vi "Actor Core.vi"(8 "error in":errorcluster, 11 "TestSetup in":refnum<class "TestSetup.lvclass">) -> (0 "error out":errorcluster, 3 "Actor out":refnum<class "Actor.lvclass">)   [LabVIEW 2019, in "TestSetup.lvlib" / "TestSetup.lvclass"]
doc: "(<B>Filename</B>: Actor Framework.lvlib:Actor.lvclass:Actor Core.vi)\n\nReceives messages to the actor, reacts to them, and initiates any error handling that may shut the actor down.\n\nDescendant classes may override this VI to append parallel tasks for the actor to complete while it handles messages. Overrides use the Call Parent Method node."
uses:
  TestSetup.lvclass
  C:/Program Files (x86)/National Instruments/LabVIEW 2019/vi.lib/ActorFramework/Actor/Actor.lvclass
  <vilib>/ActorFramework/Actor/Actor.lvclass
  TestSetup.lvclass/TestSetup.ctl
  <vilib>/ActorFramework/Actor/Actor.lvclass/Actor.ctl
  <vilib>/ActorFramework/Message Enqueuer/Message Enqueuer.lvclass/Message Enqueuer.ctl
  TestSetup Messages/LimitSetting Msg/LimitSetting Msg.lvclass/LimitSetting Msg.ctl
  226a1422-65c0-414f-be6e-00db8bf823a7.vi
  <vilib>/ActorFramework/Message Enqueuer/Init from Existing Queue.vi
  <vilib>/ActorFramework/Message Enqueuer/Enqueue.vi
  SystemSetup/SystemSetup Messages/RefreshSystemConfigurationUI Msg/RefreshSystemConfigurationUI Msg.lvclass
  C:/Program Files (x86)/National Instruments/LabVIEW 2019/vi.lib/ActorFramework/Message/Message.lvclass
  SystemSetup/SystemSetup Messages/SaveSystemConfigurationUI Msg/SaveSystemConfigurationUI Msg.lvclass
  TestSetup Messages/LimitSetting Msg/LimitSetting Msg.lvclass
  <vilib>/ActorFramework/Message Priority Queue/Priority Enqueue.vi
  <vilib>/ActorFramework/Message Enqueuer/Message Enqueuer.lvclass
  SystemSetup/SystemSetup/SystemSetup.lvclass
panel:
  in  "Multicolumn Listbox":i32(listbox)
  in  "Refresh":bool
  in  "TestLimitPath":path
  in  "Save":bool
  in  "Cancel":bool
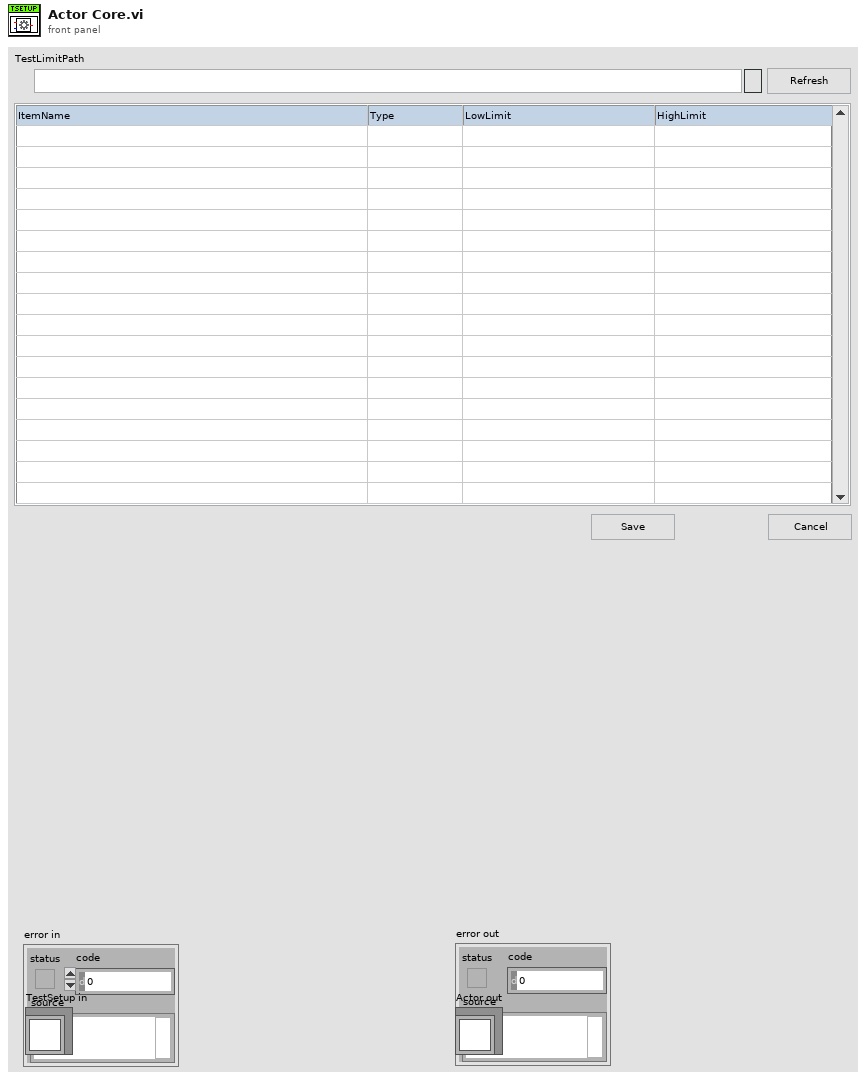
[diagram p1: front panel]
types:
  T1 = enum32{"existing file", "new file", "new or existing file", "existing dir", "new dir", "new or existing dir", "existing file (use LLBs)", "new file (use LLBs)", "new or existing file (use LLBs)", "new or existing file or directory (use LLBs)", "existing dir (use LLBs)", "new dir (use LLBs)", "new or existing dir (use LLBs)", "existing file or dir", "new file or dir", "new or existing file or dir", "existing file or dir (use LLBs)", "new file or dir (use LLBs)"}
  T2 = enum32{"Invalid", "Standard", "Closed", "Hidden", "Minimized", "Maximized"}
  T3 = enum32{"invalid app kind", "Development System", "Run Time System", "Student Edition", "Embedded LabVIEW", "Evaluation", "Custom"}
  T4 = cluster{"Core":cluster{"Current VI Reference":refnum<vi>, "Close Panel on Exit?":bool}, "Your Boolean data":bool, "Your string data":string}
  T5 = cluster{"Current VI Reference":refnum<vi>, "Close Panel on Exit?":bool}
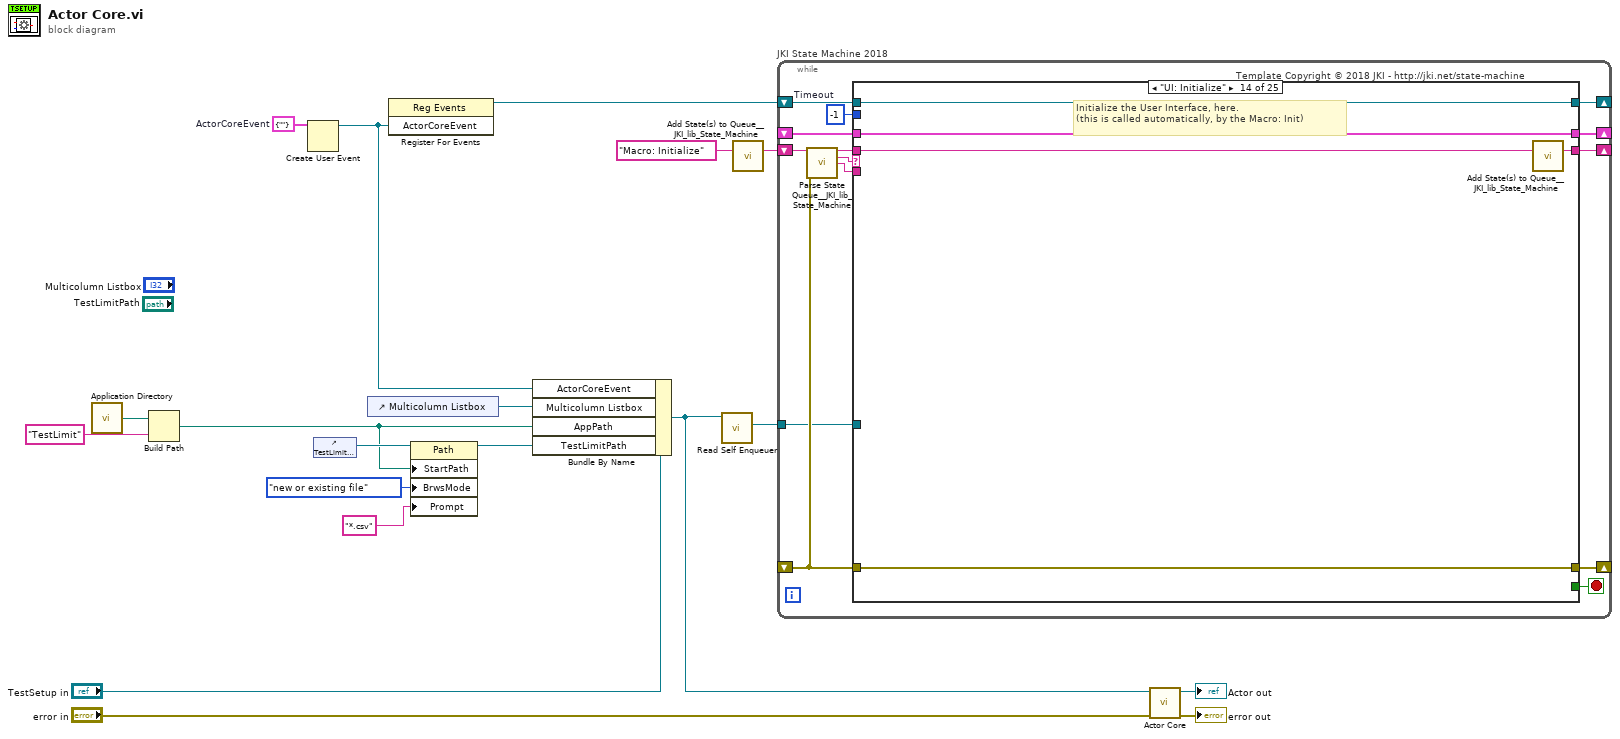
[diagram p0: block diagram]
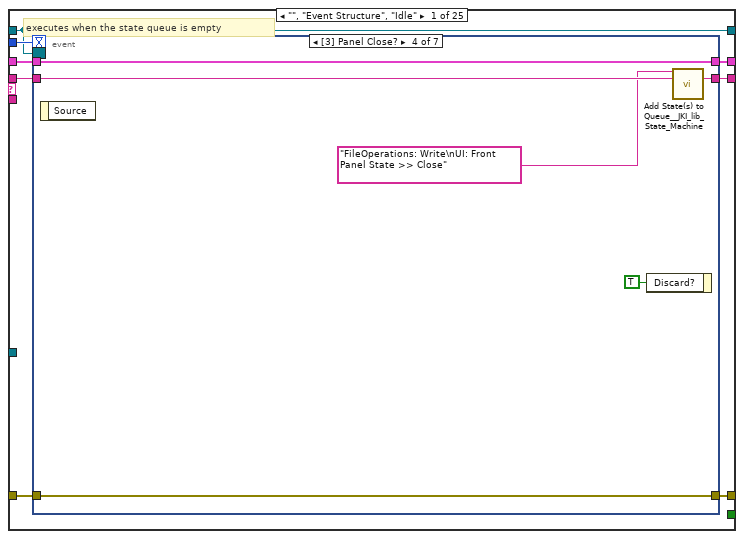
[diagram p2: hidden frame]
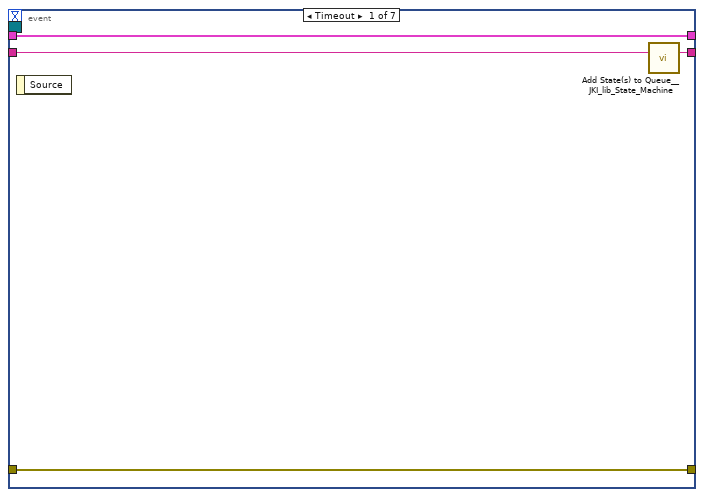
[diagram p3: hidden frame]
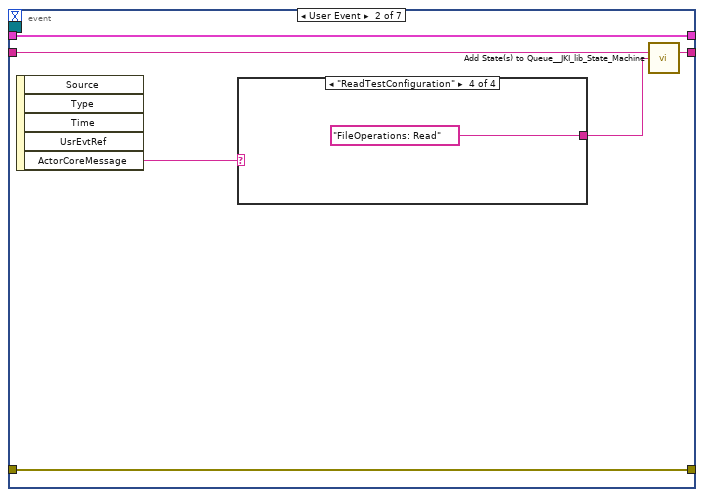
[diagram p4: hidden frame]
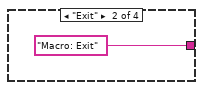
[diagram p6: hidden frame]
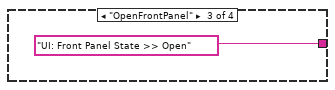
[diagram p7: hidden frame]
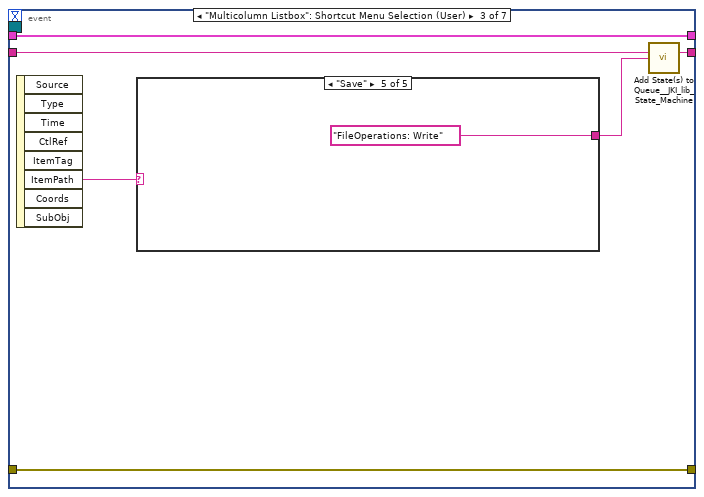
[diagram p8: hidden frame]
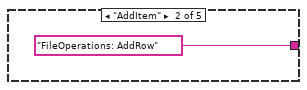
[diagram p10: hidden frame]
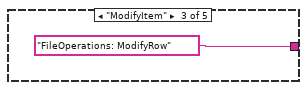
[diagram p11: hidden frame]
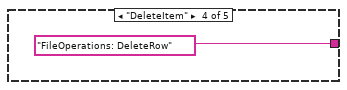
[diagram p12: hidden frame]
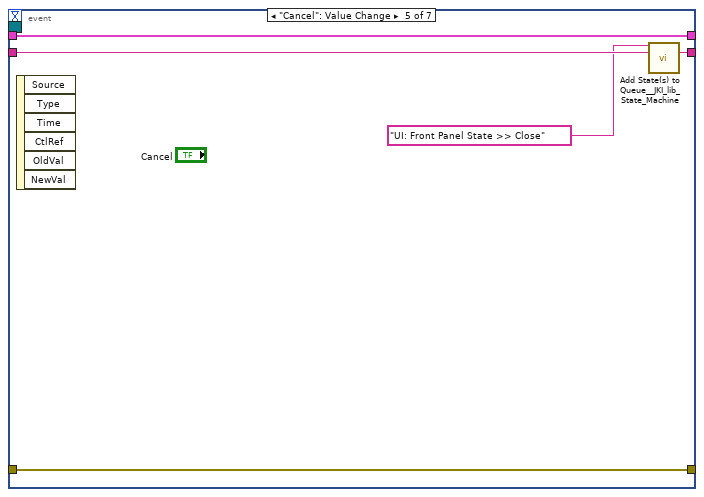
[diagram p13: hidden frame]
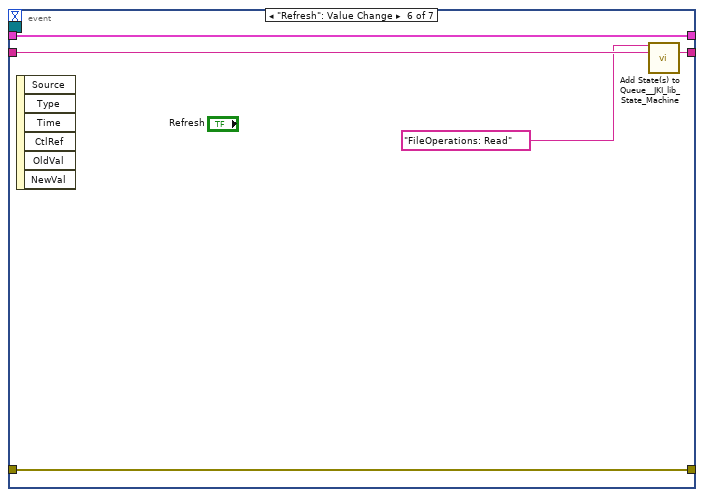
[diagram p14: hidden frame]
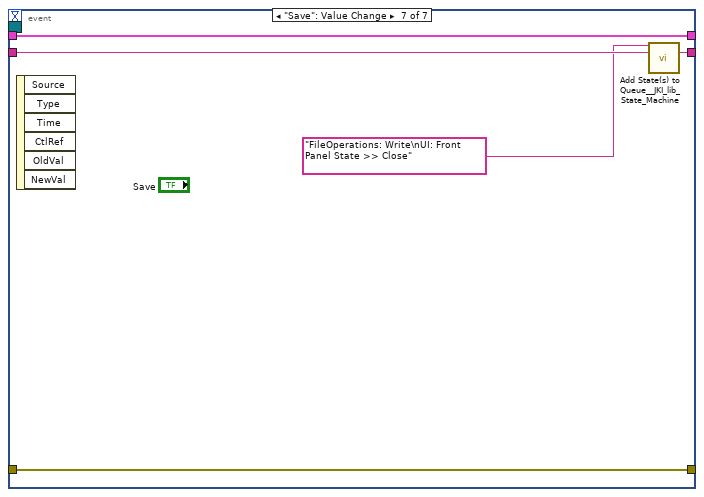
[diagram p15: hidden frame]
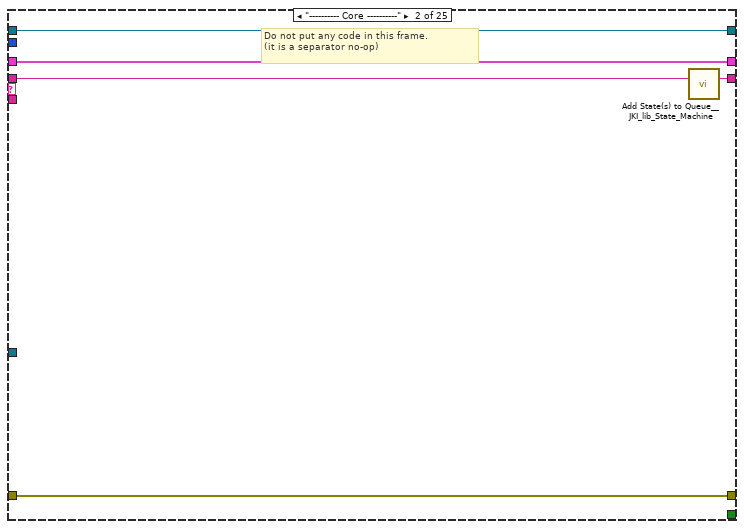
[diagram p16: hidden frame]
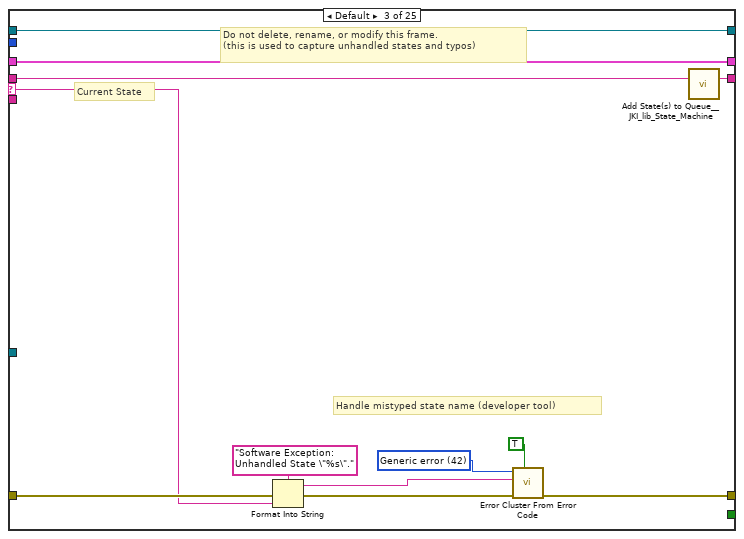
[diagram p17: hidden frame]
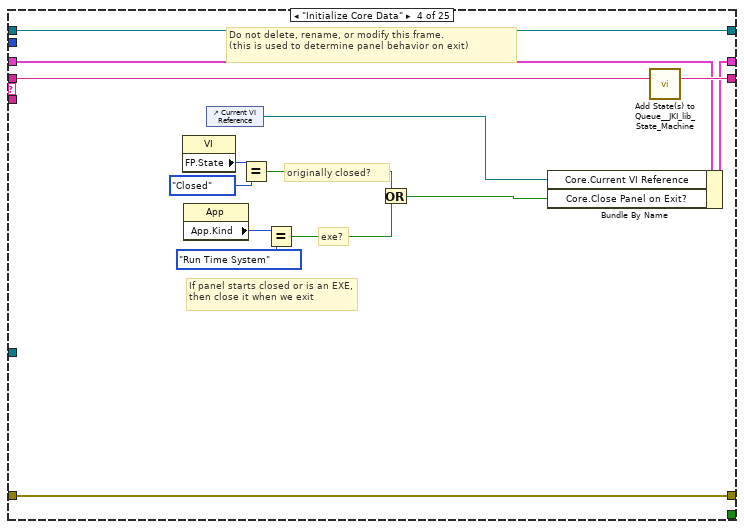
[diagram p18: hidden frame]
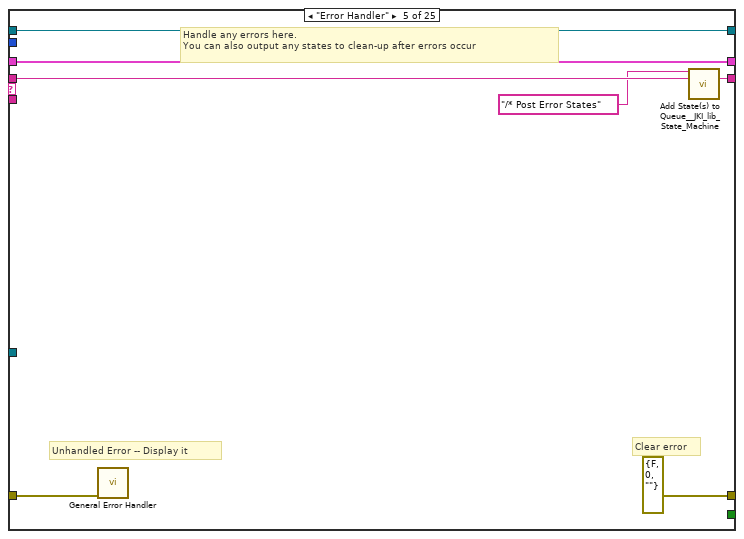
[diagram p19: hidden frame]
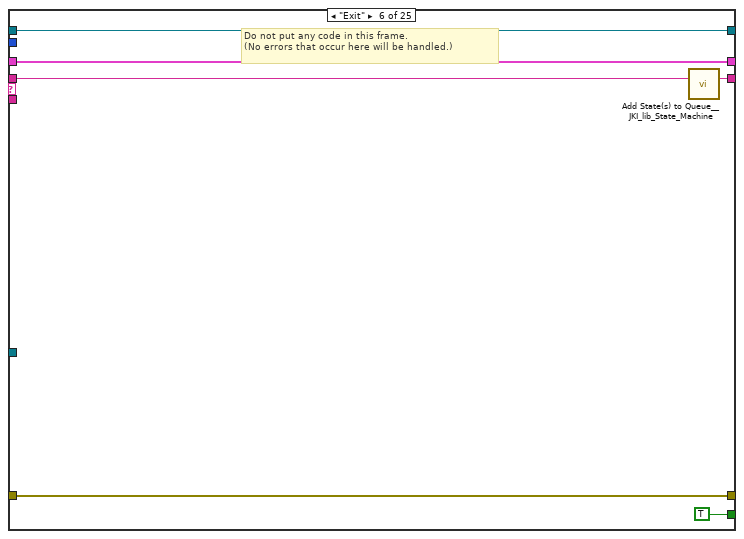
[diagram p20: hidden frame]
diagram:
  w13 = cluster{"ActorCoreMessage":string} {"ActorCoreMessage"=""}  # ActorCoreEvent
  n1 = call <vilib>:"Application Directory.vi"() -> ("Application Directory"=w7:path)
  n2 = Build Path(base path=w7, name or relative path="TestLimit") -> (appended path=w4:path)
  n3 = Create User Event(user event datatype=w13) -> (user event=w11:refnum<user-event>)  [unwired: 1 in, 1 out]
  n4 = control-ref of="TestLimitPath"() -> (w6:refnum<vi>)
  n5 = control-ref of="Multicolumn Listbox"() -> (w1:refnum<vi>)
  n6 = register-events(w11) -> (reference out=w14:refnum<event-registration>)  [unwired: 2 in, 1 out]
  n7 = property class="Path"(reference=w6, "StartPath"=w4, "BrwsMode"=T1."new or existing file" ("Browse Options:Selection Mode"), "Prompt"="*.csv" ("Browse Options:Pattern Label")) -> (reference out=w5:refnum<vi>)  [unwired: 1 in, 1 out]
  n8 = Bundle By Name(cluster="TestSetup in", "ActorCoreEvent"=w11, "Multicolumn Listbox"=w1, "AppPath"=w4, "TestLimitPath"=w5) -> (w10:refnum<class "TestSetup.lvclass">)
  n9 = call <vilib>:"Read Self Enqueuer.vi"("Actor"=w10) -> ("Self Enqueuer"=w9:refnum<class "Message Enqueuer.lvclass">)  [unwired: 10 in]
  n10 = call <vilib>:"Add State(s) to Queue__JKI_lib_State_Machine.vi"("State(s) in (\"\")"="Macro: Initialize") -> ("States Out"=w16:string)  [unwired: 14 in]
  n11 = while "JKI State Machine 2018" {
    shift-right: [w26] -> _
    shift-left: _ -> [w25]
    shift-right: [w29] -> _
    shift-left: _ -> [w23]
    shift-right: [w28] -> _
    shift-left: w16 -> [w30]
    shift-right: [w22] -> _
    shift-left: w14 -> [w21]
    tunnel: w9 -> [w20]
    stop <- w27 stop-if-true
    w24 = -1  # Timeout
    # "Template Copyright © 2018 JKI - http://jki.net/state-machine"
    n12 = call <vilib>:"Parse State Queue__JKI_lib_State_Machine.vi"("State Queue"=w30, "Error In (no error)"=w23) -> ("Remaining States"=w32:string, "Current State"=w33:string, "Arguments"=w31:string)  [unwired: 11 in]
    n13 = case shown="\"UI: Initialize\"" w33 {
      selector: w33 -> [_ _ w92 _ _ _ _ _ _ _ _ _ _ _ _ _ _ _ _ _ _ _ _ _ _]
      tunnel: w32 -> [w41 w90 w96 w116 w123 w129 w134 w142 w149 w154 w159 w165 w170 w175 w182 w194 w264 w272 w283 w288 w294 w300 w307 w314 w321]
      tunnel: w31 -> [_ _ _ _ _ _ _ _ _ _ _ _ _ _ w177 w188 _ _ _ _ _ _ _ _ _]
      tunnel: w25 -> [w39 w87 w94 w109 w120 w127 w131 _ w144 w151 w157 w163 w167 w172 w180 w190 w261 w269 w280 w285 w290 w296 w303 w310 w317]
      tunnel: [w38 w88 w98 w113 errorcluster {"status"=FALSE, "code"=0, "source"=""} ("error out") w126 w132 w139 w145 w152 w156 w160 w168 w171 w178 w191 w262 w266 w281 w286 w292 w298 w305 w312 w319] -> w29
      tunnel: w23 -> [w37 w88 w97 w113 w119 w126 w132 w139 w146 w152 w156 w161 w168 w171 w179 w192 w262 w270 w281 w286 w292 w298 w305 w312 w319]
      tunnel: [w40 w89 w95 w115 w122 w128 w133 w141 w148 w153 w158 w164 w169 w174 w181 w193 w263 w271 w282 w287 w293 w299 w306 w313 w320] -> w28
      tunnel: [_ _ _ _ _ TRUE _ _ _ _ _ _ _ _ _ _ _ _ _ _ _ _ _ _ _] -> w27
      tunnel: [w36 w87 w94 w114 w120 w127 w131 w140 w144 w151 w157 w163 w167 w172 w180 w190 w261 w269 w280 w285 w290 w296 w303 w310 w317] -> w26
      tunnel: w24 -> [w35 _ _ _ _ _ _ _ _ _ _ _ _ _ _ _ _ _ _ _ _ _ _ _ _]
      tunnel: [w34 w86 w91 w103 w117 w124 w130 w135 w143 w150 w155 w162 w166 w173 w176 w187 w260 w267 w273 w284 w291 w297 w304 w311 w318] -> w22
      tunnel: w21 -> [w34 w86 w91 w103 w117 w124 w130 w135 w143 w150 w155 w162 w166 w173 w176 w187 w260 w267 w273 w284 w291 w297 w304 w311 w318]
      tunnel: w20 -> [_ _ _ _ _ _ _ _ _ _ _ _ _ _ _ _ _ _ _ _ w289 w295 w302 w308 w315]
      frame "", "Event Structure", "Idle" {
        # "executes when the state queue is empty"
        n14 = event shown="[3] Panel Close?" {
          selector: w34 -> [_ _ _ _ _ _ _]
          dyn-events: _ -> [_ _ _ _ _ _ _]
          timeout: w35 -> [_ _ _ _ _ _ _]
          tunnel: w41 -> [w45 w51 w60 w70 w75 w80 w85]
          tunnel: [w44 w50 w59 w69 w74 w79 w84] -> w40
          tunnel: w39 -> [w42 w48 w57 w67 w72 w77 w82]
          tunnel: [w43 w49 w58 w68 w73 w78 w83] -> w38
          tunnel: w37 -> [w43 w49 w58 w68 w73 w78 w83]
          tunnel: [w42 w48 w57 w67 w72 w77 w82] -> w36
          event Timeout {
            n15 = event-data() -> ()  [unwired: 1 in, 1 out]
            n16 = call <vilib>:"Add State(s) to Queue__JKI_lib_State_Machine.vi"("State(s) in (\"\")"=w45) -> ("States Out"=w44:string)  [unwired: 14 in]
          }
          event User Event {
            n17 = event-data() -> ("ActorCoreMessage"=w47:string)  [unwired: 1 in, 4 out]
            n18 = case shown="\"ReadTestConfiguration\"" w47 {
              tunnel: [_ "Macro: Exit" "UI: Front Panel State >> Open" "FileOperations: Read"] -> w46
              frame "Idle", Default {
              }
              frame "Exit" {
              }
              frame "OpenFrontPanel" {
              }
              frame "ReadTestConfiguration" {
              }
            }
            n19 = call <vilib>:"Add State(s) to Queue__JKI_lib_State_Machine.vi"("State(s) in (\"\")"=w51, "State(s) at Back (\"\")"=w46) -> ("States Out"=w50:string)  [unwired: 13 in]
          }
          event "Multicolumn Listbox": Shortcut Menu Selection (User) {
            n20 = event-data() -> ("ItemPath"=w55:string)  [unwired: 1 in, 7 out]
            n21 = case shown="\"Save\"" w55 {
              tunnel: [_ "FileOperations: AddRow" "FileOperations: ModifyRow" "FileOperations: DeleteRow" "FileOperations: Write"] -> w56
              frame "Idle", Default {
              }
              frame "AddItem" {
              }
              frame "ModifyItem" {
              }
              frame "DeleteItem" {
              }
              frame "Save" {
              }
            }
            n22 = call <vilib>:"Add State(s) to Queue__JKI_lib_State_Machine.vi"("State(s) in (\"\")"=w60, "State(s) at Back (\"\")"=w56) -> ("States Out"=w59:string)  [unwired: 13 in]
          }
          event Panel Close? {
            n23 = event-data() -> ()  [unwired: 1 in, 1 out]
            n24 = event-data("Discard?"=TRUE) -> ()  [unwired: 1 in, 1 out]
            n25 = call <vilib>:"Add State(s) to Queue__JKI_lib_State_Machine.vi"("State(s) in Front (\"\")"="FileOperations: Write\nUI: Front Panel State >> Close", "State(s) in (\"\")"=w70) -> ("States Out"=w69:string)  [unwired: 13 in]
          }
          event "Cancel": Value Change {
            n26 = event-data() -> ()  [unwired: 1 in, 6 out]
            n27 = call <vilib>:"Add State(s) to Queue__JKI_lib_State_Machine.vi"("State(s) in Front (\"\")"="UI: Front Panel State >> Close", "State(s) in (\"\")"=w75) -> ("States Out"=w74:string)  [unwired: 13 in]
          }
          event "Refresh": Value Change {
            n28 = event-data() -> ()  [unwired: 1 in, 6 out]
            n29 = call <vilib>:"Add State(s) to Queue__JKI_lib_State_Machine.vi"("State(s) in Front (\"\")"="FileOperations: Read", "State(s) in (\"\")"=w80) -> ("States Out"=w79:string)  [unwired: 13 in]
          }
          event "Save": Value Change {
            n30 = event-data() -> ()  [unwired: 1 in, 6 out]
            n31 = call <vilib>:"Add State(s) to Queue__JKI_lib_State_Machine.vi"("State(s) in Front (\"\")"="FileOperations: Write\nUI: Front Panel State >> Close", "State(s) in (\"\")"=w85) -> ("States Out"=w84:string)  [unwired: 13 in]
          }
        }
      }
      frame "---------- Core ----------" {
        # "Do not put any code in this frame.\n(it is a separator no-op)"
        n32 = call <vilib>:"Add State(s) to Queue__JKI_lib_State_Machine.vi"("State(s) in (\"\")"=w90) -> ("States Out"=w89:string)  [unwired: 14 in]
      }
      frame Default {
        w101 = 42 items=["No error", "Argument error", "Memory is full", "Out of zone", "End of file", "File already open", "Generic file I/O error", "File not found", "File permission error", "Disk is full", "Duplicate path", "Too many files open", "System feature not enabled", "Resource file not found", "Cannot add resource", "Resource not found", "Image not found", "Image memory error", "Pen does not exist", "Config type invalid", "Config token not found", "Config parse error", "Config memory error", "Bad external code format", "Bad external code offset", "External code not present", "Null window", "Destroy window error", "Null menu", "Print aborted", "Bad print record", "Print driver error", "Windows error during printing", "Memory error during printing", "Print dialog error", "Generic print error", "Invalid device refnum", "Device not found", "Device parameter error", "Device unit error", "Cannot open device", "Device call aborted", "Generic error", "Cancelled by user", "Object ID too low", "Object ID too high", "Object not in heap", "Unknown heap", "Unknown object (invalid DefProc)", "Unknown object (DefProc not in table)", "Message out of range", "Invalid (null) method", "Unknown message", "Manager call not supported", "Bad address", "Network operation in progress", "Network operation timed out", "Connection is busy", "Network attribute not supported", "Network error", "Address in use", "System out of memory", "Connection aborted", "Connection refused", "Not connected", "Already connected", "Connection closed", "Initialization error (interapplication manager)", "Bad occurrence", "Wait on unbound occurrence handler", "Occurrence queue overflow", "Datalog type conflict", "Unused", "Unrecognized type (interapplication manager)", "Memory corrupt", "Failed to make temporary DLL", "Old CIN version", "Drag socket not found", "Failed to load drop-object", "Failed to register OLE object", "Failed to release OLE object", "Format specifier type mismatch", "Unknown format specifier", "Too few format specifiers", "Too many format specifiers", "Scan failed", "Newer CIN version", "Error converting to variant", "Runtime menu error", "Password tampered", "Variant attribute not found", "Incompatible variant data type", "Event data is not available", "Event Store is not present", "Occurrence is not found", "Event Queue is not created", "Event info is not available", "Refnum passed is NULL", "Error retrieving Class GUID", "Error retrieving CoClass GUID", "Error retrieving TypeLib GUID.", "Bad built application magic bytes.", "Specific driver is different from the specific driver associated with the Logical Name.", "There is no session opened to the class driver.", "Max Error", "MAX - Error with config objects", "MAX - Error loading configuration", "MAX - Group not supported"]
        # "Current State"
        # "Do not delete, rename, or modify this frame.\n(this is used to capture unhandled states and typos)"
        # "Handle mistyped state name (developer tool)"
        n33 = Format Into String(format string="Software Exception: Unhandled State \"%s\"." ("message"), error in=w97, w92) -> (resulting string=w100:string, error out=w99:errorcluster)  [unwired: 1 in]
        n34 = call <vilib>:"Error Cluster From Error Code.vi"("show call chain? (False)"=TRUE, "error in (no error)"=w99, "error message (\"\")"=w100, "error code (0)"=w101) -> ("error out"=w98:errorcluster)  [unwired: 5 in]
        n35 = call <vilib>:"Add State(s) to Queue__JKI_lib_State_Machine.vi"("State(s) in (\"\")"=w96) -> ("States Out"=w95:string)  [unwired: 14 in]
      }
      frame "Initialize Core Data" {
        # "Do not delete, rename, or modify this frame.\n(this is used to determine panel behavior on exit)"
        # "originally closed?"
        # "exe?"
        # "If panel starts closed or is an EXE, then close it when we exit"
        n36 = property class="VI"() -> ("FP.State"=w106:T2)  [unwired: 2 in, 2 out]
        n37 = property class="App"() -> ("App.Kind"=w112:T3)  [unwired: 2 in, 2 out]
        n38 = control-ref of="Current VI Reference"() -> (w107:refnum<vi>)
        n39 = Equal?(x=w106, y=T2."Closed" ("Front Panel Window:State")) -> (x = y?=w104:bool)
        n40 = Equal?(x=w112, y=T3."Run Time System" ("Application:Kind")) -> (x = y?=w110:bool)
        n41 = Or(x=w104, y=w110) -> (x .or. y?=w108:bool)
        n42 = Bundle By Name(cluster=w109, "Core.Current VI Reference"=w107, "Core.Close Panel on Exit?"=w108) -> (w114:T4)
        n43 = call <vilib>:"Add State(s) to Queue__JKI_lib_State_Machine.vi"("State(s) in (\"\")"=w116) -> ("States Out"=w115:string)  [unwired: 14 in]
      }
      frame "Error Handler" {
        # "Unhandled Error -- Display it"
        # "Handle any errors here.\nYou can also output any states to clean-up after errors occur"
        # "Clear error"
        n44 = call <vilib>:"General Error Handler.vi"("error in (no error)"=w119) -> ()  [unwired: 10 in, 5 out]
        n45 = call <vilib>:"Add State(s) to Queue__JKI_lib_State_Machine.vi"("State(s) in Front (\"\")"="/* Post Error States", "State(s) in (\"\")"=w123) -> ("States Out"=w122:string)  [unwired: 13 in]
      }
      frame "Exit" {
        # "Do not put any code in this frame.\n(No errors that occur here will be handled.)"
        n46 = call <vilib>:"Add State(s) to Queue__JKI_lib_State_Machine.vi"("State(s) in (\"\")"=w129) -> ("States Out"=w128:string)  [unwired: 14 in]
      }
      frame "---------- Data ----------" {
        # "Do not put any code in this frame.\n(It is a separator no-op. You can make a copy of this frame to create a new Data frame)"
        n47 = call <vilib>:"Add State(s) to Queue__JKI_lib_State_Machine.vi"("State(s) in (\"\")"=w134) -> ("States Out"=w133:string)  [unwired: 14 in]
      }
      frame "Data: Initialize" {
        w136 = T5 {"Current VI Reference"=refnum, "Close Panel on Exit?"=FALSE}  # Core
        w138 = TRUE  # Your Boolean data
        w137 = ""  # Your string data
        # "Data names and types of shift register data are defined by this bundle."
        # "Initialize the shift-register data, here.\n(data names are defined by what you wire into the bundle function)"
        n48 = Bundle("Core"=w136, "Your Boolean data"=w138, "Your string data"=w137) -> (w140:T4)  [unwired: 1 in]
        n49 = call <vilib>:"Add State(s) to Queue__JKI_lib_State_Machine.vi"("State(s) in (\"\")"=w142) -> ("States Out"=w141:string)  [unwired: 14 in]
      }
      frame "Data: Cleanup" {
        # "Cleanup any data and references, here.\n(this is called automatically, by the Macro: Exit)"
        n50 = Unbundle By Name(w144) -> ("Core.Current VI Reference"=w147:refnum<vi>)
        n51 = Close Reference(reference=w147, error in (no error)=w146) -> (error out=w145:errorcluster)
        n52 = call <vilib>:"Add State(s) to Queue__JKI_lib_State_Machine.vi"("State(s) in (\"\")"=w149) -> ("States Out"=w148:string)  [unwired: 14 in]
      }
      frame "---------- Events ----------" {
        # "Do not put any code in this frame.\n(It is a separator no-op. You can make a copy of this frame to create a new UI frame)"
        n53 = call <vilib>:"Add State(s) to Queue__JKI_lib_State_Machine.vi"("State(s) in (\"\")"=w154) -> ("States Out"=w153:string)  [unwired: 14 in]
      }
      frame "Events: Register" {
        n54 = call <vilib>:"Add State(s) to Queue__JKI_lib_State_Machine.vi"("State(s) in (\"\")"=w159) -> ("States Out"=w158:string)  [unwired: 14 in]
      }
      frame "Events: Unregister" {
        # "Do not put any code in this frame.\n(It is a separator no-op. You can make a copy of this frame to create a new UI frame)"
        n55 = Unregister For Events(event registration refnum=w162, error in=w161) -> (error out=w160:errorcluster)
        n56 = call <vilib>:"Add State(s) to Queue__JKI_lib_State_Machine.vi"("State(s) in (\"\")"=w165) -> ("States Out"=w164:string)  [unwired: 14 in]
      }
      frame "---------- UI ----------" {
        # "Do not put any code in this frame.\n(It is a separator no-op. You can make a copy of this frame to create a new UI frame)"
        n57 = call <vilib>:"Add State(s) to Queue__JKI_lib_State_Machine.vi"("State(s) in (\"\")"=w170) -> ("States Out"=w169:string)  [unwired: 14 in]
      }
      frame "UI: Initialize" {
        # "Initialize the User Interface, here.\n(this is called automatically, by the Macro: Init)"
        n58 = call <vilib>:"Add State(s) to Queue__JKI_lib_State_Machine.vi"("State(s) in (\"\")"=w175) -> ("States Out"=w174:string)  [unwired: 14 in]
      }
      frame "UI: Cursor Set" {
        # "Argument"
        # "Set and Unset Cursor Busy.\n(Usage: \"UI: Cursor Set >> Busy|Idle\")"
        n59 = case shown="\"Idle\", Default" w177 {
          tunnel: w179 -> [w184 w186]
          tunnel: [w183 w185] -> w178
          frame "Idle", Default {
            n60 = call <vilib>:"Unset Busy.vi"("error in (no error)"=w184) -> ("error out"=w183:errorcluster)  [unwired: 10 in]
          }
          frame "Busy" {
            n61 = call <vilib>:"Set Busy.vi"("error in (no error)"=w186) -> ("error out"=w185:errorcluster)  [unwired: 9 in, 1 out]
          }
        }
        n62 = call <vilib>:"Add State(s) to Queue__JKI_lib_State_Machine.vi"("State(s) in (\"\")"=w182) -> ("States Out"=w181:string)  [unwired: 14 in]
      }
      frame "UI: Front Panel State" {
        # "Argument"
        # "Set Front Panel Open or Closed\n(Usage: \"UI: Front Panel State >> Open|Close\")"
        n63 = Unbundle By Name(w190) -> ("Core.Current VI Reference"=w189:refnum<vi>)
        n64 = case shown="\"Minimize\", \"Minimized\"" w188 {
          tunnel: w192 -> [w200 w215 w226 w239 w252]
          tunnel: [w202 w216 w228 w241 w254] -> w191
          tunnel: w189 -> [w201 w213 w227 w240 w253]
          frame "Open", "Standard", Default {
            w195 = T2."Standard" ("State")
            n65 = property class="VI"(reference=w201, error in=w200) -> (reference out=w198:refnum<vi>, error out=w199:errorcluster, "FP.State"=w197:T2)
            n66 = Not Equal?(x=w197, y=w195) -> (x != y?=w196:bool)
            n67 = case shown="True" w196 {
              tunnel: [w206 w208] -> w202
              tunnel: w199 -> [w205 w208]
              tunnel: w198 -> [w204 _]
              tunnel: w195 -> [w203 _]
              frame True {
                n68 = invoke class="VI" method="FP.Open"(reference=w204, error in=w205, "Activate"=TRUE, "State"=w203) -> (error out=w206:errorcluster)  [unwired: 1 in, 4 out]
              }
              frame False {
              }
            }
          }
          frame "Close", "Closed" {
            n69 = property class="VI"(reference=w213, error in=w215) -> (reference out=w212:refnum<vi>, error out=w214:errorcluster, "FP.State"=w210:T2)
            n70 = Not Equal?(x=w210, y=T2."Closed" ("Front Panel Window:State")) -> (x != y?=w209:bool)
            n71 = case shown="True" w209 {
              tunnel: [w217 w220] -> w216
              tunnel: w214 -> [w217 w219]
              tunnel: w212 -> [_ w218]
              frame False {
              }
              frame True {
                n72 = invoke class="VI" method="FP.Close"(reference=w218, error in=w219) -> (error out=w220:errorcluster)  [unwired: 1 in, 2 out]
              }
            }
          }
          frame "Hidden", "Hide" {
            w221 = T2."Hidden" ("State")
            n73 = property class="VI"(reference=w227, error in=w226) -> (reference out=w224:refnum<vi>, error out=w225:errorcluster, "FP.State"=w223:T2)
            n74 = Not Equal?(x=w223, y=w221) -> (x != y?=w222:bool)
            n75 = case shown="True" w222 {
              tunnel: [w232 w233] -> w228
              tunnel: w225 -> [w231 w233]
              tunnel: w224 -> [w230 _]
              tunnel: w221 -> [w229 _]
              frame True {
                n76 = invoke class="VI" method="FP.Open"(reference=w230, error in=w231, "State"=w229) -> (error out=w232:errorcluster)  [unwired: 2 in, 4 out]
              }
              frame False {
              }
            }
          }
          frame "Minimize", "Minimized" {
            w234 = T2."Minimized" ("State")
            n77 = property class="VI"(reference=w240, error in=w239) -> (reference out=w237:refnum<vi>, error out=w238:errorcluster, "FP.State"=w236:T2)
            n78 = Not Equal?(x=w236, y=w234) -> (x != y?=w235:bool)
            n79 = case shown="True" w235 {
              tunnel: [w245 w246] -> w241
              tunnel: w238 -> [w244 w246]
              tunnel: w237 -> [w243 _]
              tunnel: w234 -> [w242 _]
              frame True {
                n80 = invoke class="VI" method="FP.Open"(reference=w243, error in=w244, "State"=w242) -> (error out=w245:errorcluster)  [unwired: 2 in, 4 out]
              }
              frame False {
              }
            }
          }
          frame "Maximize", "Maximized" {
            w247 = T2."Maximized" ("State")
            n81 = property class="VI"(reference=w253, error in=w252) -> (reference out=w250:refnum<vi>, error out=w251:errorcluster, "FP.State"=w249:T2)
            n82 = Not Equal?(x=w249, y=w247) -> (x != y?=w248:bool)
            n83 = case shown="True" w248 {
              tunnel: [w258 w259] -> w254
              tunnel: w251 -> [w257 w259]
              tunnel: w250 -> [w256 _]
              tunnel: w247 -> [w255 _]
              frame True {
                n84 = invoke class="VI" method="FP.Open"(reference=w256, error in=w257, "State"=w255) -> (error out=w258:errorcluster)  [unwired: 2 in, 4 out]
              }
              frame False {
              }
            }
          }
        }
        n85 = call <vilib>:"Add State(s) to Queue__JKI_lib_State_Machine.vi"("State(s) in (\"\")"=w194) -> ("States Out"=w193:string)  [unwired: 14 in]
      }
      frame "---------- Macro ----------" {
        # "Do not put any code in this frame.\n(It is a separator no-op. You can make a copy of this frame to create a new Macro frame)"
        n86 = call <vilib>:"Add State(s) to Queue__JKI_lib_State_Machine.vi"("State(s) in (\"\")"=w264) -> ("States Out"=w263:string)  [unwired: 14 in]
      }
      frame "Macro: Initialize" {
        # "Initialization Macro\n(This is called once, when the VI starts)"
        n87 = call "Stall Data Flow.vim"("value in"=w270, "milliseconds to wait"=u32 500) -> ("value out"=w266:errorcluster)  [unwired: 1 out]
        n88 = call <vilib>:"Add State(s) to Queue__JKI_lib_State_Machine.vi"("State(s) in Front (\"\")"="Data: Initialize\nInitialize Core Data\nEvents: Register\nUI: Initialize\nUI: Front Panel State >> Close", "State(s) in (\"\")"=w272) -> ("States Out"=w271:string)  [unwired: 13 in]
      }
      frame "Macro: Exit" {
        # "Exit Macro\n(This is called once, when the VI exits)"
        n89 = Unbundle By Name(w280) -> ("Core.Close Panel on Exit?"=w279:bool)
        n90 = Select(t="UI: Front Panel State >> Close", s=w279, f="") -> (s? t:f=w276:string)
        n91 = call <vilib>:"Add State(s) to Queue__JKI_lib_State_Machine.vi"("State(s) in (\"\")"=w276, "State(s) at Back (\"\")"="Data: Cleanup\nEvents: Unregister\nExit") -> ("States Out"=w274:string)  [unwired: 13 in]
        n92 = call <vilib>:"Add State(s) to Queue__JKI_lib_State_Machine.vi"("State(s) in Front (\"\")"=w274, "State(s) in (\"\")"=w283) -> ("States Out"=w282:string)  [unwired: 13 in]
      }
      frame "---------- FileOperations ----------" {
        # "Template Separator\n(You can make a copy of, or modify, this frame)"
        n93 = call <vilib>:"Add State(s) to Queue__JKI_lib_State_Machine.vi"("State(s) in (\"\")"=w288) -> ("States Out"=w287:string)  [unwired: 14 in]
      }
      frame "FileOperations: Read" {
        # "Your code here.\n(You can make a copy of, or modify, this frame)"
        n94 = call "Send RefreshSystemConfigurationUI.vi"("Message Enqueuer"=w289) -> ()  [unwired: 9 in, 2 out]
        n95 = call <vilib>:"Add State(s) to Queue__JKI_lib_State_Machine.vi"("State(s) in (\"\")"=w294) -> ("States Out"=w293:string)  [unwired: 14 in]
      }
      frame "FileOperations: Write" {
        # "Your code here.\n(You can make a copy of, or modify, this frame)"
        n96 = call "Send SaveSystemConfigurationUI.vi"("Message Enqueuer"=w295) -> ()  [unwired: 9 in, 2 out]
        n97 = call <vilib>:"Add State(s) to Queue__JKI_lib_State_Machine.vi"("State(s) in (\"\")"=w300) -> ("States Out"=w299:string)  [unwired: 14 in]
      }
      frame "FileOperations: AddRow" {
        # "Your code here.\n(You can make a copy of, or modify, this frame)"
        n98 = call "Send LimitSetting.vi"("operation"=enum16{"Add", "Delete", "Modify"}."Add", "Message Enqueuer"=w302) -> ()  [unwired: 8 in, 2 out]
        n99 = call <vilib>:"Add State(s) to Queue__JKI_lib_State_Machine.vi"("State(s) in (\"\")"=w307) -> ("States Out"=w306:string)  [unwired: 14 in]
      }
      frame "FileOperations: ModifyRow" {
        # "Your code here.\n(You can make a copy of, or modify, this frame)"
        n100 = call "Send LimitSetting.vi"("operation"=enum16{"Add", "Delete", "Modify"}."Modify", "Message Enqueuer"=w308) -> ()  [unwired: 8 in, 2 out]
        n101 = call <vilib>:"Add State(s) to Queue__JKI_lib_State_Machine.vi"("State(s) in (\"\")"=w314) -> ("States Out"=w313:string)  [unwired: 14 in]
      }
      frame "FileOperations: DeleteRow" {
        # "Your code here.\n(You can make a copy of, or modify, this frame)"
        n102 = call "Send LimitSetting.vi"("operation"=enum16{"Add", "Delete", "Modify"}."Delete", "Message Enqueuer"=w315) -> ()  [unwired: 8 in, 2 out]
        n103 = call <vilib>:"Add State(s) to Queue__JKI_lib_State_Machine.vi"("State(s) in (\"\")"=w321) -> ("States Out"=w320:string)  [unwired: 14 in]
      }
    }
  }
  n104 = call-parent "Actor Core.vi"("error in"="error in", "Actor in"=w10) -> ("error out"=→"error out":errorcluster, "Actor out"=→"Actor out":refnum<class "Actor.lvclass">)  [unwired: 8 in]
